vi "thermalCamera.vi"() -> ()   [LabVIEW 2025]
panel:
  out "IP address":string
  in  "Stop Button":bool
  out "Output":string
  in  "Flag":bool
  in  "Stop recording":bool
  in  "Stop Preview":bool
  in  "Server Path":path
  in  "Focus":dbl(slide) scale=0.0..100.0
  in  "Record":bool
  in  "Connect Server":bool
  out "?":string
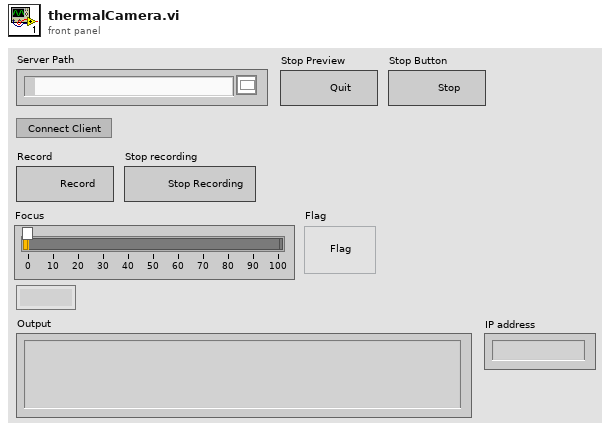
[diagram p1: front panel]
types:
  T1 = enum16{"Standard", "Buffered", "CRLF", "Immediate"}
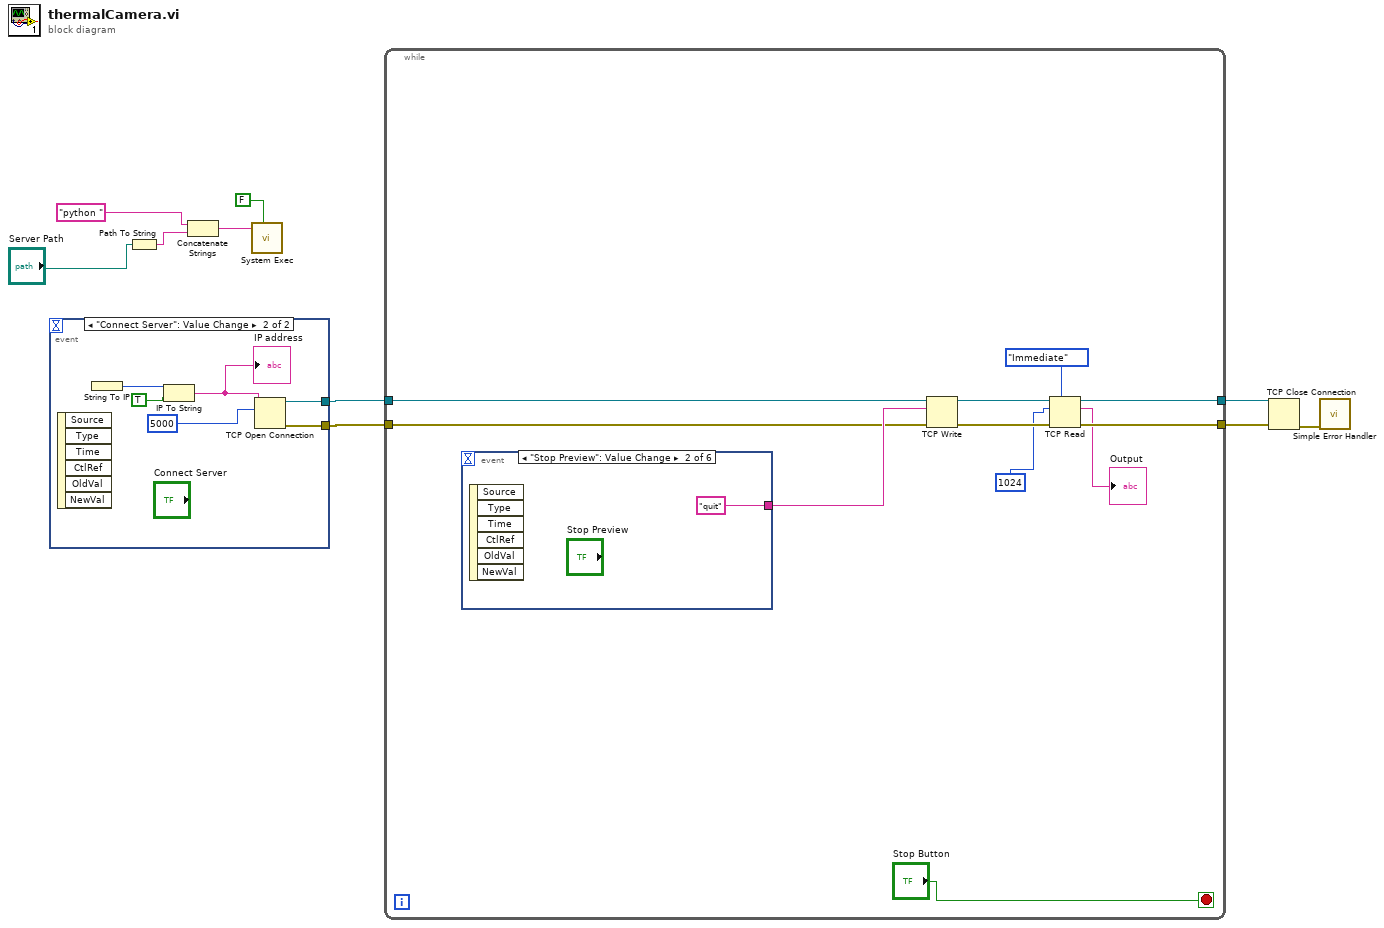
[diagram p0: block diagram]
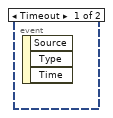
[diagram p2: hidden frame]
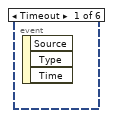
[diagram p3: hidden frame]
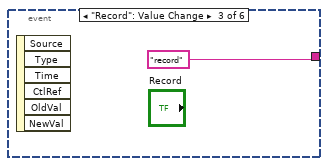
[diagram p4: hidden frame]
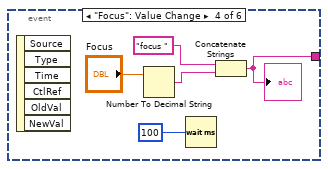
[diagram p5: hidden frame]
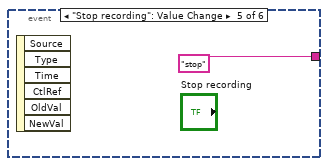
[diagram p6: hidden frame]
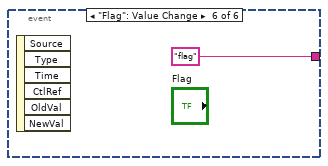
[diagram p7: hidden frame]
diagram:
  n1 = event shown="[1] \"Connect Server\": Value Change" {
    selector: _ -> [_ _]
    dyn-events: _ -> [_ _]
    timeout: _ -> [_ _]
    tunnel: [_ w15] -> w5
    tunnel: [_ w14] -> w4
    event Timeout {
      n2 = event-data() -> ()  [unwired: 1 in, 3 out]
    }
    event "Connect Server": Value Change {
      n3 = event-data() -> ()  [unwired: 1 in, 6 out]
      n4 = String To IP() -> (0:w13:u32)  [unwired: 1 in]
      n5 = IP To String(1:TRUE ("dot notation? (F)"), 2:w13) -> (0:w11:string)
      "IP address" <- w11
      n6 = TCP Open Connection(address=w11, remote port or service name=u16 5000) -> (connection ID=w14:refnum<k5>, error out=w15:errorcluster)  [unwired: 3 in]
    }
  }
  n7 = Path To String(path="Server Path") -> (string=w6:string)
  n8 = Concatenate Strings("python " ("string"), w6) -> (w2:string)
  n9 = call <vilib>:"System Exec.vi"("wait until completion? (T)"=FALSE, "command line"=w2) -> ()  [unwired: 6 in, 4 out]
  n10 = while {
    tunnel: [w26] -> w10
    tunnel: [w24] -> w9
    tunnel: w5 -> [w22]
    tunnel: w4 -> [w21]
    stop <- "Stop Button" stop-if-true
    n11 = event shown="[1] \"Stop Preview\": Value Change" {
      selector: _ -> [_ _ _ _ _ _]
      dyn-events: _ -> [_ _ _ _ _ _]
      timeout: _ -> [_ _ _ _ _ _]
      tunnel: [_ "quit" "record" w32 "stop" "flag"] -> w23
      event Timeout {
        n12 = event-data() -> ()  [unwired: 1 in, 3 out]
      }
      event "Stop Preview": Value Change {
        n13 = event-data() -> ()  [unwired: 1 in, 6 out]
      }
      event "Record": Value Change {
        n14 = event-data() -> ()  [unwired: 1 in, 6 out]
      }
      event "Focus": Value Change {
        n15 = event-data() -> ()  [unwired: 1 in, 6 out]
        n16 = Number To Decimal String(number="Focus") -> (decimal integer string=w34:string)  [unwired: 1 in]
        n17 = Wait (ms)(milliseconds to wait=u32 100) -> ()  [unwired: 1 out]
        n18 = Concatenate Strings("focus ", w34) -> (w32:string)
        "?" <- w32
      }
      event "Stop recording": Value Change {
        n19 = event-data() -> ()  [unwired: 1 in, 6 out]
      }
      event "Flag": Value Change {
        n20 = event-data() -> ()  [unwired: 1 in, 6 out]
      }
    }
    n21 = TCP Write(connection ID=w21, data in=w23, error in (no error)=w22) -> (connection ID out=w25:refnum<k5>, error out=w27:errorcluster)  [unwired: 1 in, 1 out]
    n22 = TCP Read(connection ID=w25, bytes to read=1024, error in (no error)=w27, 7:T1."Immediate" ("mode (standard)")) -> (connection ID out=w24:refnum<k5>, data out=→"Output":string, error out=w26:errorcluster)  [unwired: 1 in]
  }
  n23 = TCP Close Connection(connection ID=w9, error in (no error)=w10) -> (error out=w8:errorcluster)  [unwired: 1 in, 1 out]
  n24 = call <vilib>:"Simple Error Handler.vi"("error in (no error)"=w8) -> ()  [unwired: 4 in, 5 out]
